vi "CSM - Check If Module Exists.vi"(8 "Error in":errorcluster caption="Error in (no error)", 11 "CSM Name":string) -> (0 "Error out":errorcluster, 2 "Exist?":bool, 3 "CSM Name(dup)":string)   [LabVIEW 2020, in "Communicable State Machine.lvlib"]
doc: "Check if module with specified name exists.\n\n<b>Inputs:</b>\n - <b>CSM Name</b>: CSM Module Name\n - <b>Error in</b>: Error cluster\n\n<b>Outputs:</b>\n - <b>Exist?</b>: Return True if spcified module exists.\n - <b>CSM Name(dup)</b>: Return <b>CSM Name</b>\n - <b>Error out</b>: Error cluster"
uses:
  Communicable State Machine.lvlib
  Priority Queue.lvclass/Priority Queue.ctl
  Obtain Priority Queue.vi
  Priority Queue.lvclass
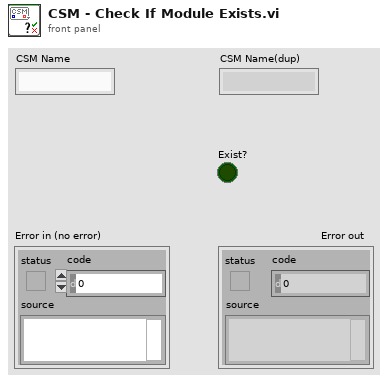
[diagram p1: front panel]
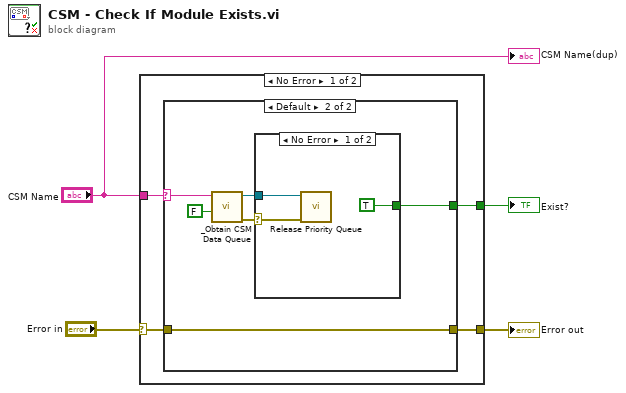
[diagram p0: block diagram]
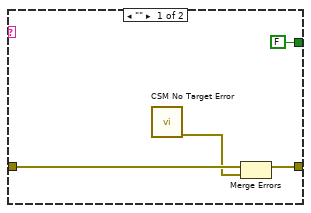
[diagram p2: hidden frame]
diagram:
  n1 = case shown="No Error" "Error in" {
    selector: "Error in" -> [w5 w22]
    tunnel: "CSM Name" -> [w8 _]
    tunnel: [w7 _] -> w3
    tunnel: [w6 w22] -> w1
    frame No Error {
      n2 = case shown="Default" w8 {
        selector: w8 -> [_ w18]
        tunnel: [FALSE w14] -> w7
        tunnel: [w10 w13] -> w6
        tunnel: w5 -> [w11 w13]
        frame "" {
          n3 = call "CSM No Target Error.vi"() -> ("error out"=w9:errorcluster)  [unwired: 11 in]
          n4 = Merge Errors(w11, w9) -> (w10:errorcluster)
        }
        frame Default {
          n5 = call "_Obtain CSM Data Queue.vi"("create if not found? (T)"=FALSE, "Name"=w18) -> ("error out"=w16:errorcluster, "Priority Queue"=w15:refnum<class "Priority Queue.lvclass">)  [unwired: 7 in, 1 out]
          n6 = case shown="No Error" w16 {
            selector: w16 -> [w20 _]
            tunnel: w15 -> [w21 _]
            tunnel: [TRUE _] -> w14
            frame No Error {
              n7 = call "Release Priority Queue.vi"("error in (no error)"=w20, "Priority Queue"=w21) -> ()  [unwired: 9 in, 1 out]
            }
            frame Error {
            }
          }
        }
      }
    }
    frame Error {
    }
  }
  "Error out" <- w1
  "Exist?" <- w3
  "CSM Name(dup)" <- "CSM Name"
